vi "ProcessTemplate (Minimal).vi"   [LabVIEW 2013]
uses:
  SMO/SMO.lvclass
  SMO/Typedefs/Parent Call--Enum.ctl
types:
  T1 = typedef "SMO.lvclass/Parent Call--Enum.ctl" = enum16{"Allows parent to run", "Does not request parent to run"}
  T2 = typedef "SMO.lvclass/Protected Events.ctl" = cluster{"StopProcesses":refnum<user-event>, "AbortProcesses":refnum<user-event>, "Config Changed":refnum<user-event>, "Dependency":refnum<user-event>}
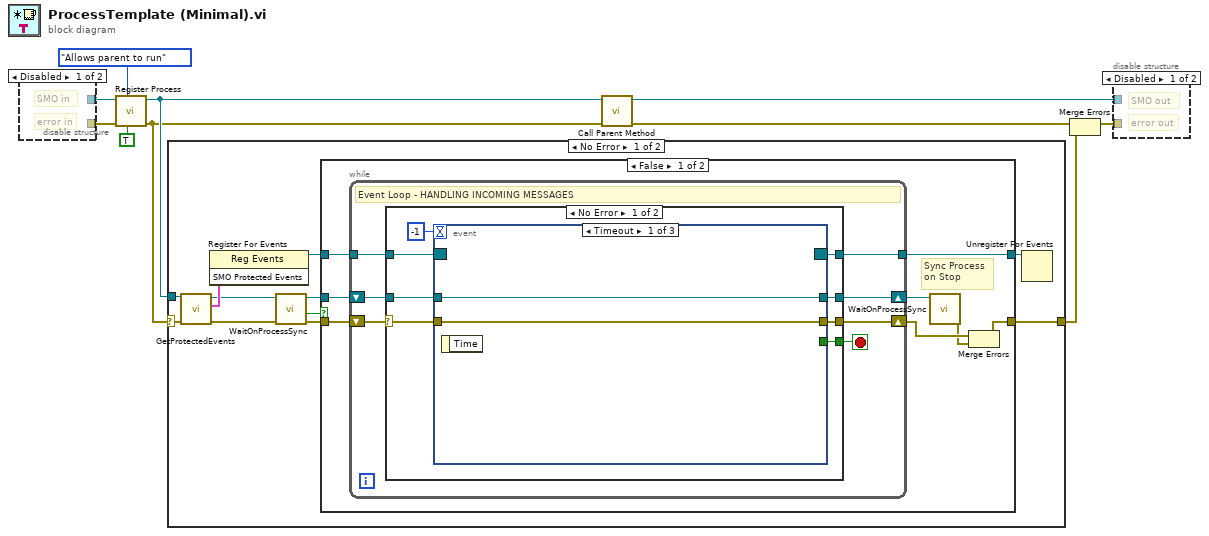
[diagram p0: block diagram]
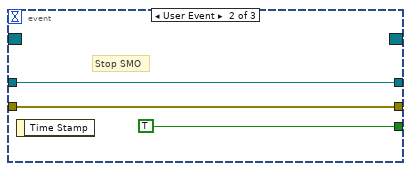
[diagram p4: hidden frame]
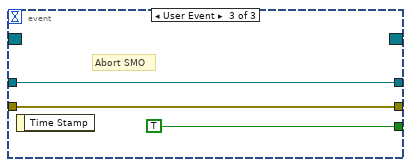
[diagram p5: hidden frame]
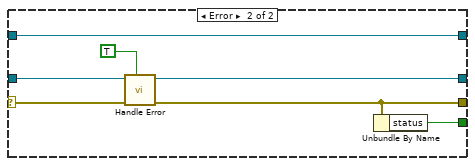
[diagram p6: hidden frame]
diagram:
  n1 = disable-structure shown="Disabled" {
    disable-tunnel: w3 -> [_ _]
    disable-tunnel: [_ _] -> w2
    frame Disabled {
      # "error in"
      # "SMO in"
    }
    frame Enabled {
    }
  }
  n2 = call "Register Process.vi"("Forces Self to Run (F)"=TRUE, "Parent Call"=Parent_Call--Enum."Allows parent to run", "error in (no error)"=w2) -> ("error out"=w9:errorcluster, "SMO out"=w10:refnum<class "SMO.lvclass">, "SMO"=w3:refnum<class "SMO.lvclass">)  [unwired: 6 in]
  n3 = case shown="No Error" w9 {
    selector: w9 -> [w17 w62]
    tunnel: w10 -> [w20 _]
    tunnel: [w13 w62] -> w6
    frame No Error {
      n4 = call "GetProtectedEvents.vi"("error in (no error)"=w17, "SMO"=w20) -> ("error out"=w18:errorcluster, "SMO Protected Events"=w21:T2, "SMO out"=w19:refnum<class "SMO.lvclass">)  [unwired: 7 in]
      n5 = register-events(w21) -> (reference out=w11:refnum<event-registration>)  [unwired: 2 in, 1 out]
      n6 = call "WaitOnProcessSync.vi"("error in (no error)"=w18, "SMO"=w19) -> ("error out"=w15:errorcluster, "Don't run?"=w14:bool, "SMO out"=w16:refnum<class "SMO.lvclass">)  [unwired: 7 in]
      n7 = case shown="False" w14 {
        tunnel: w15 -> [w25 w60]
        tunnel: w16 -> [w27 _]
        tunnel: w11 -> [w29 w61]
        tunnel: [w22 w60] -> w13
        tunnel: [w28 w61] -> w12
        frame False {
          # "Sync Process\non Stop"
          n8 = while {
            tunnel: w29 -> [w36]
            tunnel: [w35] -> w28
            shift-right: [w32] -> w26
            shift-left: w27 -> [w33]
            shift-right: [w31] -> w24
            shift-left: w25 -> [w30]
            stop <- w34 stop-if-true
            # "Event Loop - HANDLING INCOMING MESSAGES"
            n9 = case shown="No Error" w30 {
              selector: w30 -> [w37 w57]
              tunnel: w36 -> [w43 w59]
              tunnel: [w42 w59] -> w35
              tunnel: [w41 w53] -> w34
              tunnel: w33 -> [w40 w56]
              tunnel: [w39 w55] -> w32
              tunnel: [w38 w54] -> w31
              frame No Error {
                n10 = event shown="[0] Timeout" {
                  selector: w43 -> [_ _ _]
                  dyn-events: [_ _ _] -> w42
                  timeout: -1 -> [_ _ _]
                  tunnel: [_ TRUE TRUE] -> w41
                  tunnel: w40 -> [w46 w48 w51]
                  tunnel: [w46 w48 w51] -> w39
                  tunnel: [w45 w47 w50] -> w38
                  tunnel: w37 -> [w45 w47 w50]
                  event Timeout {
                    n11 = event-data() -> ()  [unwired: 1 in, 1 out]
                  }
                  event User Event {
                    # "Stop SMO"
                    n12 = event-data() -> ()  [unwired: 1 in, 1 out]
                  }
                  event User Event {
                    # "Abort SMO"
                    n13 = event-data() -> ()  [unwired: 1 in, 1 out]
                  }
                }
              }
              frame Error {
                n14 = call-dynamic "Handle Error.vi"("Stop on Unhandled Error (T)"=TRUE, "error in"=w57, "SMO"=w56) -> ("handling error"=w54:errorcluster, "SMO out"=w55:refnum<class "SMO.lvclass">)  [unwired: 6 in, 1 out]
                n15 = Unbundle By Name(w54) -> ("status"=w53:bool)
              }
            }
          }
          n16 = call "WaitOnProcessSync.vi"("SMO"=w26) -> ("error out"=w23:errorcluster)  [unwired: 8 in, 2 out]
          n17 = Merge Errors(w24, w23) -> (w22:errorcluster)
        }
        frame True {
        }
      }
      n18 = Unregister For Events(event registration refnum=w12) -> ()  [unwired: 1 in, 1 out]
    }
    frame Error {
    }
  }
  n19 = call-parent "Call Parent Method"("error in"=w9, "SMO"=w10) -> ("error out"=w8:errorcluster, "SMO out"=w4:refnum<class "SMO.UI.lvclass">)  [unwired: 8 in]
  n20 = Merge Errors(w8, w6) -> (w5:errorcluster)
  n21 = disable-structure shown="Disabled" {
    disable-tunnel: w5 -> [_ _]
    disable-tunnel: w4 -> [_ _]
    frame Disabled {
      # "error out"
      # "SMO out"
    }
    frame Enabled {
    }
  }
